vi "Draw Glyph.vi"(5 "Transform (Center)":refnum<class "Transform.lvclass">, 6 "Colors":T1={"Front"={"Color"=0, "Alpha"=255}, "Back"={"Color"=16777215, "Alpha"=255}}, 7 "Font (System)":refnum<class "Font Settings.lvclass">, 8 "error in (no error)":errorcluster, 9 "Destination":refnum<class "Glyph Canvas.lvclass">, 10 "codepoint":u32 format="%.0x", 11 "Canvas .Net in":refnum<class "Drawer .Net.lvclass">) -> (0 "error out":errorcluster, 1 "Glyph Canvas out":refnum<class "Glyph Canvas.lvclass">, 3 "Canvas .Net out":refnum<class "Drawer .Net.lvclass">)   [LabVIEW 2023, in "Glyph .NET.lvlib" / "Drawer .Net.lvclass"]
uses:
  Drawer .Net.lvclass
  Font Glyph Drawer Interface/Glyph Canvas/Glyph Canvas.lvclass
  Font Glyph Drawer Interface/Font Settings/Font Settings.lvclass
  Font Glyph Drawer Interface/Transform/Transform.lvclass
  System.Drawing
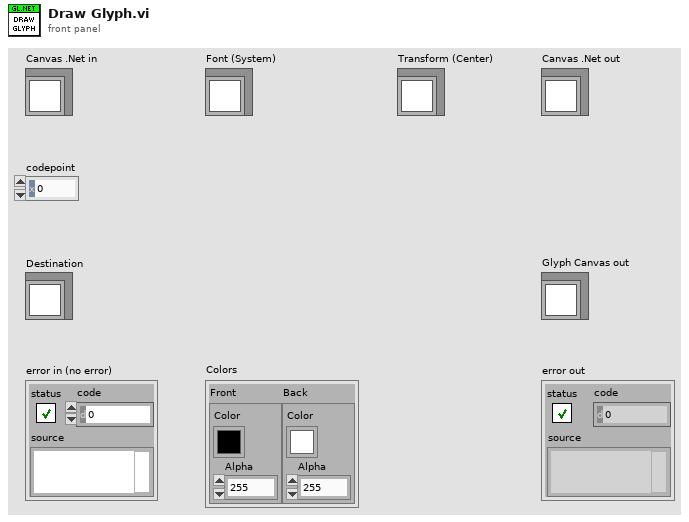
[diagram p1: front panel]
types:
  T1 = cluster{"Front":cluster{"Color":u32, "Alpha":u8}, "Back":cluster{"Color":u32, "Alpha":u8}}
  T2 = typedef "NI_Matrix.lvlib/RealMatrix.ctl" = dbl[][]
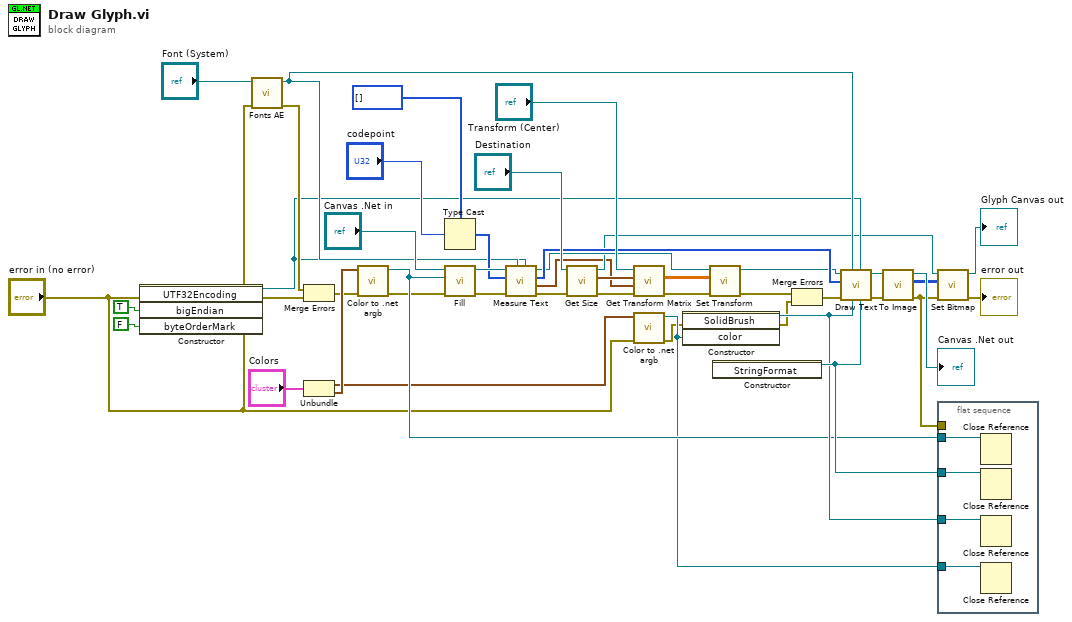
[diagram p0: block diagram]
diagram:
  n1 = constructor class="UTF32Encoding"(error in="error in (no error)", "bigEndian"=TRUE, "byteOrderMark"=FALSE) -> (reference out=w16:refnum<k24>, error out=w39:errorcluster)  [unwired: 2 in, 3 out]
  n2 = call "Fonts AE.vi"("error in (no error)"="error in (no error)", "Font"="Font (System)") -> ("error out"=w35:errorcluster, "Font"=w17:refnum<k24>)  [unwired: 8 in]
  n3 = Merge Errors(w35, w39) -> (w9:errorcluster)
  n4 = Unbundle("Colors") -> ("Front"=w27:cluster{"Color":u32, "Alpha":u8}, "Back"=w29:cluster{"Color":u32, "Alpha":u8})
  n5 = call "Color to .net argb.vi"("error in (no error)"=w9, "Color"=w29) -> ("error out"=w8:errorcluster, "FromArgb"=w28:refnum<k24>)  [unwired: 8 in]
  n6 = Type Cast(type=u8[] [], x="codepoint") -> (*(type *) &x=w18:u8[])
  n7 = call "Fill.vi"("error in (no error)"=w8, "Color"=w28, "Canvas in"="Canvas .Net in") -> ("error out"=w34:errorcluster, "Canvas out"=w19:refnum<class "Drawer .Net.lvclass">)  [unwired: 7 in]
  n8 = call "Measure Text.vi"("Encoding"=w16, "Font"=w17, "error in (no error)"=w34, "Text Raw"=w18, "Canvas in"=w19) -> ("error out"=w20:errorcluster, "Size"=w3:cluster{"Width":sgl, "Height":sgl}, "Text Raw"=w15:u8[], "Canvas out"=w13:refnum<class "Drawer .Net.lvclass">)  [unwired: 3 in]
  n9 = call-dynamic "Get Size.vi"("error in (no error)"=w20, "Glyph Destination in"="Destination") -> ("error out"=w4:errorcluster, "Size"=w21:cluster{"Width":u16, "Height":u16}, "Glyph Destination out"=w12:refnum<class "Glyph Canvas.lvclass">)  [unwired: 7 in]
  n10 = call-dynamic "Get Transform Matrix.vi"("error in (no error)"=w4, "Glyph Size"=w3, "Canvas Size"=w21, "Transform in"="Transform (Center)") -> ("error out"=w2:errorcluster, "Transform"=w1:T2)  [unwired: 5 in, 1 out]
  n11 = call "Color to .net argb.vi"("error in (no error)"="error in (no error)", "Color"=w27) -> ("error out"=w11:errorcluster, "FromArgb"=w26:refnum<k24>)  [unwired: 8 in]
  n12 = constructor class="SolidBrush"(error in=w11, "color"=w26) -> (reference out=w30:refnum<k24>, error out=w10:errorcluster)  [unwired: 2 in, 2 out]
  n13 = call "Set Transform.vi"("error in (no error)"=w2, "Real Matrix 2x3"=w1, "Drawer .Net in"=w13) -> ("error out"=w6:errorcluster, "Drawer .Net out"=w14:refnum<class "Drawer .Net.lvclass">)  [unwired: 7 in]
  n14 = constructor class="StringFormat"() -> (reference out=w37:refnum<k24>)  [unwired: 3 in, 2 out]
  n15 = Merge Errors(w6, w10) -> (w7:errorcluster)
  n16 = call "Draw Text.vi"("Text Format"=w37, "Encoding"=w16, "Brush"=w30, "Font"=w17, "error in (no error)"=w7, "Bytes"=w15, "Canvas in"=w14) -> ("error out"=w43:errorcluster, "Canvas out"=w45:refnum<class "Drawer .Net.lvclass">)  [unwired: 3 in]
  n17 = call "To Image.vi"("error in (no error)"=w43, "Canvas in"=w45) -> ("error out"=w36:errorcluster, "Bitmap"=w42:u32[][], "Canvas out"=→"Canvas .Net out":refnum<class "Drawer .Net.lvclass">)  [unwired: 7 in]
  n18 = call-dynamic "Set Bitmap.vi"("error in (no error)"=w36, "Bitmap"=w42, "Glyph Canvas in"=w12) -> ("error out"=→"error out":errorcluster, "Glyph Canvas out"=→"Glyph Canvas out":refnum<class "Glyph Canvas.lvclass">)  [unwired: 7 in]
  n19 = flat-sequence {
    tunnel: w36 -> [_]
    tunnel: w30 -> [w50]
    tunnel: w37 -> [w49]
    tunnel: w28 -> [w48]
    tunnel: w26 -> [w47]
    frame #0 {
      n20 = Close Reference(reference=w48) -> ()  [unwired: 1 in, 1 out]
      n21 = Close Reference(reference=w49) -> ()  [unwired: 1 in, 1 out]
      n22 = Close Reference(reference=w50) -> ()  [unwired: 1 in, 1 out]
      n23 = Close Reference(reference=w47) -> ()  [unwired: 1 in, 1 out]
    }
  }
